vi "DSF.Engine.Transceiver Thread.Initialize.vi"(8 "error in (no error)":errorcluster, 11 "Transceiver Thread in":refnum<class "DSF.Engine.Transceiver Thread.lvclass">) -> (0 "error out":errorcluster, 3 "Transceiver Thread out":refnum<class "DSF.Engine.Transceiver Thread.lvclass">)   [LabVIEW 2017, in "DSF.Engine.lvlib" / "DSF.Engine.Transceiver Thread.lvclass"]
uses:
  DSF.Engine.Transceiver Thread.lvclass
  DSF.Engine.Transceiver Thread.lvclass/DSF.Engine.Transceiver Thread.ctl
  Cache/DSF.Engine.Memory.Cache.lvclass
  DSF.Engine.Transceiver.lvclass
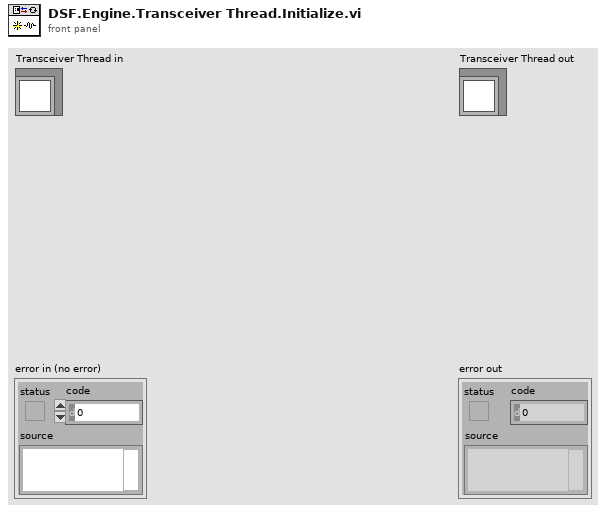
[diagram p1: front panel]
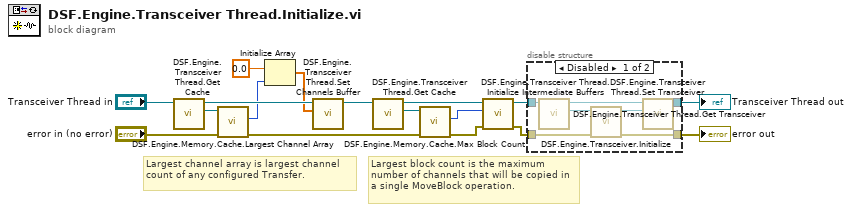
[diagram p0: block diagram]
diagram:
  # "Largest channel array is largest channel count of any configured Transfer."
  # "Largest block count is the maximum number of channels that will be copied in a single MoveBlock operation."
  n1 = call "DSF.Engine.Transceiver Thread.Get Cache.vi"("Transceiver Thread in"="Transceiver Thread in") -> ("Cache"=w15:refnum<class "DSF.Engine.Memory.Cache.lvclass">, "Transceiver Thread out"=w13:refnum<class "DSF.Engine.Transceiver Thread.lvclass">)  [unwired: 9 in]
  n2 = call "DSF.Engine.Memory.Cache.Largest Channel Array.vi"("error in (no error)"="error in (no error)", "Cache in"=w15) -> ("error out"=w8:errorcluster, "largest channel array"=w11:u64)  [unwired: 7 in, 1 out]
  n3 = Initialize Array(0.0 ("element"), w11) -> (w12:dbl[])
  n4 = call "DSF.Engine.Transceiver Thread.Set Channels Buffer.vi"("channels buffer"=w12, "Transceiver Thread in"=w13) -> ("Transceiver Thread out"=w10:refnum<class "DSF.Engine.Transceiver Thread.lvclass">)  [unwired: 9 in]
  n5 = call "DSF.Engine.Transceiver Thread.Get Cache.vi"("Transceiver Thread in"=w10) -> ("Cache"=w9:refnum<class "DSF.Engine.Memory.Cache.lvclass">, "Transceiver Thread out"=w5:refnum<class "DSF.Engine.Transceiver Thread.lvclass">)  [unwired: 9 in]
  n6 = call "DSF.Engine.Memory.Cache.Max Block Count.vi"("error in (no error)"=w8, "Cache in"=w9) -> ("error out"=w7:errorcluster, "largest block count"=w6:u64)  [unwired: 7 in, 1 out]
  n7 = call "DSF.Engine.Transceiver Thread.Initialize Intermediate Buffers.vi"("error in (no error)"=w7, "largest block count"=w6, "Transceiver Thread in"=w5) -> ("error out"=w1:errorcluster, "Transceiver Thread out"=w3:refnum<class "DSF.Engine.Transceiver Thread.lvclass">)  [unwired: 7 in]
  n8 = disable-structure shown="Disabled" {
    disable-tunnel: [w21 w25] -> w17
    disable-tunnel: [w20 w26] -> w16
    disable-tunnel: w3 -> [w19 w26]
    disable-tunnel: w1 -> [w18 w25]
    frame Disabled {
      n9 = call "DSF.Engine.Transceiver Thread.Get Transceiver.vi"("Transceiver Thread in"=w19) -> ("Transceiver"=w24:refnum<class "DSF.Engine.Transceiver.lvclass">, "Transceiver Thread out"=w22:refnum<class "DSF.Engine.Transceiver Thread.lvclass">)  [unwired: 9 in]
      n10 = call-dynamic "DSF.Engine.Transceiver.Initialize.vi"("error in (no error)"=w18, "Transceiver in"=w24) -> ("error out"=w21:errorcluster, "Transceiver out"=w23:refnum<class "DSF.Engine.Transceiver.lvclass">)  [unwired: 8 in]
      n11 = call "DSF.Engine.Transceiver Thread.Set Transceiver.vi"("Transceiver"=w23, "Transceiver Thread in"=w22) -> ("Transceiver Thread out"=w20:refnum<class "DSF.Engine.Transceiver Thread.lvclass">)  [unwired: 9 in]
    }
    frame Enabled {
    }
  }
  "error out" <- w17
  "Transceiver Thread out" <- w16
